vi "ActuatorSetup_Read_INI_local.vi"(8 "Error In":errorcluster, 11 "Config File Path":path) -> (0 "Error Out":errorcluster, 2 "Actuator setup Parameters":T1)   [LabVIEW 2017]
uses:
  <vilib>/Utility/config.llb/Read Key (I32).vi
  <vilib>/Utility/config.llb/Read Key (String).vi
  <vilib>/Utility/config.llb/Read Key (Path).vi
  <vilib>/Utility/config.llb/NI_LVConfig.lvlib
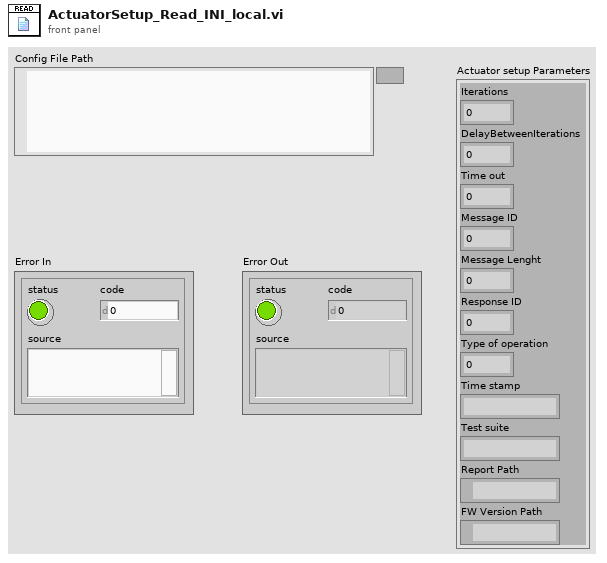
[diagram p1: front panel]
types:
  T1 = cluster{"Iterations":u64, "DelayBetweenIterations":u32, "Time out":u32, "Message ID":i32, "Message Lenght":i32, "Response ID":i32, "Type of operation":i32, "Time stamp":string, "Test suite":string, "Report Path":path, "FW Version Path":path}
  T2 = typedef "NI_LVConfig.lvlib/Config Data RefNum.ctl" = refnum<k1>
  T3 = cluster{u64, u32, u32, i32, i32, i32, "value":i32, "value":string, "value":string, "value":path, path}
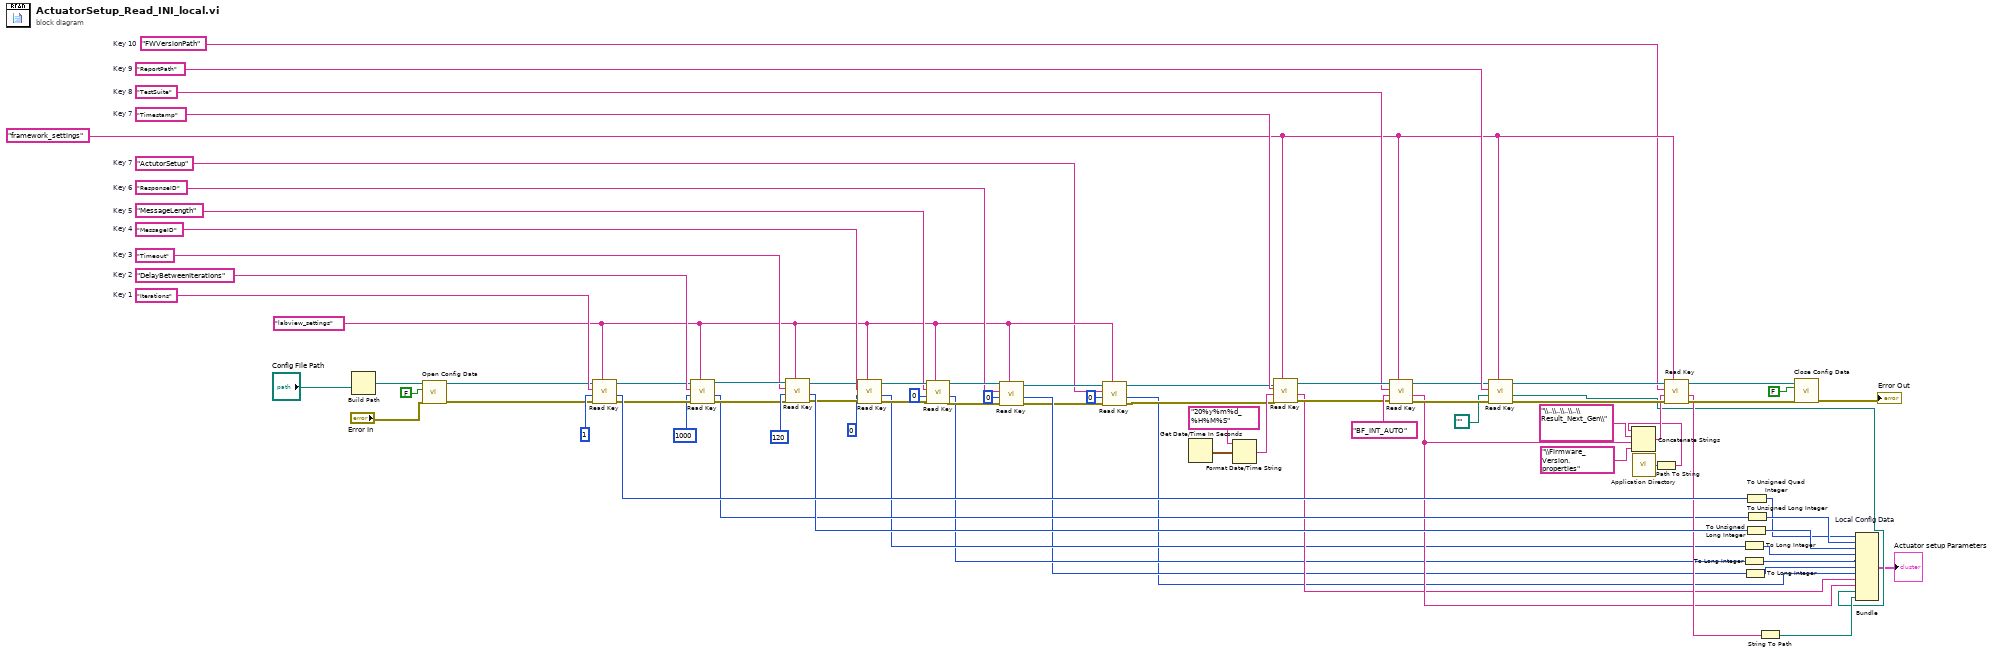
[diagram p0: block diagram]
diagram:
  w3 = "ActutorSetup"  # Key 7
  w14 = "ResponseID"  # Key 6
  w15 = "MessageLength"  # Key 5
  w33 = "MessageID"  # Key 4
  w43 = "FWVersionPath"  # Key 10
  w55 = "Timestamp"  # Key 7
  w50 = "TestSuite"  # Key 8
  w56 = "Timeout"  # Key 3
  w65 = "ReportPath"  # Key 9
  w70 = "DelayBetweenIterations"  # Key 2
  w72 = "Iterations"  # Key 1
  w44 = "framework_settings" ("section")
  w5 = "labview_settings" ("section")
  n1 = Build Path(name or relative path="Config File Path") -> (appended path=w74:path)  [unwired: 1 in]
  n2 = call <vilib>:"Open Config Data.vi"("error in (no error)"="Error In", "create file if necessary (T)"=FALSE ("create file if necessary? (T)"), "configuration file path"=w74) -> ("error out"=w36:errorcluster, "refnum"=w35:T2)  [unwired: 6 in, 1 out]
  n3 = call-poly <vilib>:"Read Key.vi"("section"=w5, "error in (no error)"=w36, "default value"=1, "key"=w72, "refnum"=w35) -> ("error out"=w68:errorcluster, "value"=w71:i32, "refnum out"=w69:T2)  [unwired: 4 out]
  n4 = call-poly <vilib>:"Read Key.vi"("section"=w5, "error in (no error)"=w68, "default value"=1000, "key"=w70, "refnum"=w69) -> ("error out"=w63:errorcluster, "value"=w34:i32, "refnum out"=w62:T2)  [unwired: 4 out]
  n5 = call-poly <vilib>:"Read Key.vi"("section"=w5, "error in (no error)"=w63, "default value"=120, "key"=w56, "refnum"=w62) -> ("error out"=w28:errorcluster, "value"=w60:i32, "refnum out"=w32:T2)  [unwired: 4 out]
  n6 = call-poly <vilib>:"Read Key.vi"("section"=w5, "error in (no error)"=w28, "default value"=0, "key"=w33, "refnum"=w32) -> ("error out"=w26:errorcluster, "value"=w21:i32, "refnum out"=w31:T2)  [unwired: 4 out]
  n7 = call-poly <vilib>:"Read Key.vi"("section"=w5, "error in (no error)"=w26, "default value"=0, "key"=w15, "refnum"=w31) -> ("error out"=w27:errorcluster, "value"=w17:i32, "refnum out"=w30:T2)  [unwired: 4 out]
  n8 = call-poly <vilib>:"Read Key.vi"("section"=w5, "error in (no error)"=w27, "default value"=0, "key"=w14, "refnum"=w30) -> ("error out"=w7:errorcluster, "value"=w16:i32, "refnum out"=w29:T2)  [unwired: 4 out]
  n9 = call-poly <vilib>:"Read Key.vi"("section"=w5, "error in (no error)"=w7, "default value"=0, "key"=w3, "refnum"=w29) -> ("error out"=w6:errorcluster, "value"=w2:i32, "refnum out"=w8:T2)  [unwired: 3 in, 1 out]
  n10 = Get Date/Time In Seconds() -> (seconds since 1Jan1904=w57:timestamp)
  n11 = Format Date/Time String(time format string (%c)="20%y%m%d_%H%M%S", seconds (now)=w57) -> (date/time string=w58:string)  [unwired: 1 out]
  n12 = call-poly <vilib>:"Read Key.vi"("section"=w44, "error in (no error)"=w6, "default value"=w58, "key"=w55, "refnum"=w8) -> ("error out"=w52:errorcluster, "value"=w22:string, "refnum out"=w53:T2)  [unwired: 1 in, 3 out]
  n13 = call-poly <vilib>:"Read Key.vi"("section"=w44, "error in (no error)"=w52, "default value"="BF_INT_AUTO", "key"=w50, "refnum"=w53) -> ("error out"=w51:errorcluster, "value"=w23:string, "refnum out"=w54:T2)  [unwired: 1 in, 3 out]
  n14 = call-poly <vilib>:"Read Key.vi"("section"=w44, "error in (no error)"=w51, "default value"=path "", "key"=w65, "refnum"=w54) -> ("error out"=w45:errorcluster, "value"=w24:path, "refnum out"=w48:T2)  [unwired: 1 in, 3 out]
  n15 = call <vilib>:"Application Directory.vi"() -> ("Application Directory"=w39:path)
  n16 = Path To String(path=w39) -> (string=w38:string)
  n17 = Concatenate Strings(w38, "\\..\\..\\..\\..\\Result_Next_Gen\\" ("default value"), w23, "\\Firmware_Version.properties" ("default value")) -> (w42:string)
  n18 = call-poly <vilib>:"Read Key.vi"("section"=w44, "error in (no error)"=w45, "default value"=w42, "key"=w43, "refnum"=w48) -> ("error out"=w46:errorcluster, "value"=w37:string, "refnum out"=w47:T2)  [unwired: 1 in, 3 out]
  n19 = To Long Integer(number=w21) -> (32bit integer=w20:i32)
  n20 = To Long Integer(number=w17) -> (32bit integer=w19:i32)
  n21 = To Long Integer(number=w16) -> (32bit integer=w18:i32)
  n22 = To Unsigned Long Integer(number=w60) -> (unsigned 32bit integer=w78:u32)
  n23 = To Unsigned Quad Integer(1:w71) -> (0:w77:u64)
  n24 = To Unsigned Long Integer(number=w34) -> (unsigned 32bit integer=w79:u32)
  n25 = String To Path(string=w37) -> (path=w25:path)
  n26 = call <vilib>:"Close Config Data.vi"("error in (no error)"=w46, "write file if changed (T)"=FALSE ("write configuration file? (T)"), "refnum"=w47) -> ("error out"=→"Error Out":errorcluster)  [unwired: 8 out]
  n27 = Bundle "Local Config Data"(w77, w79, w78, w20, w19, w18, "value"=w2, "value"=w22, "value"=w23, "value"=w24, w25) -> (→"Actuator setup Parameters":T3)  [unwired: 1 in]
